vi "Parametric or Manual Arm Movement.vi"(0 "Desired Parametric\nValue":dbl, 1 "Forearm Manual\nControl":bool=TRUE, 2 "Change in\nForearm Angle":dbl, 5 "Current Parametric\nValue":dbl, 9 "Current Backarm\nAngle":dbl, 11 "Current Forearm\nAngle":dbl, 12 "Points":dbl[][](array[numeric]), 13 "Robot\nDimensions":cluster{}) -> (4 "New Backarm\nAngle":dbl, 6 "New Forearm\nAngle":dbl, 8 "Next Parametric\nValue":dbl, 10 "Apply Backarm\nBreak":bool=TRUE, 15 "Apply Forearm\nBreak":bool=TRUE)   [LabVIEW 2017]
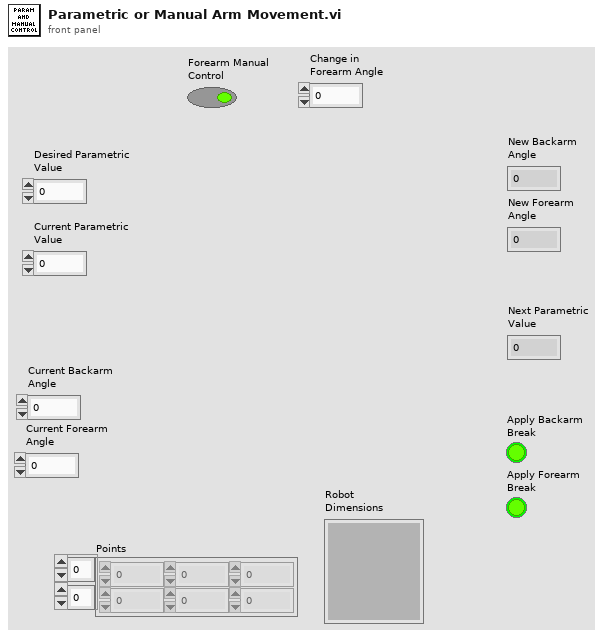
[diagram p1: front panel]
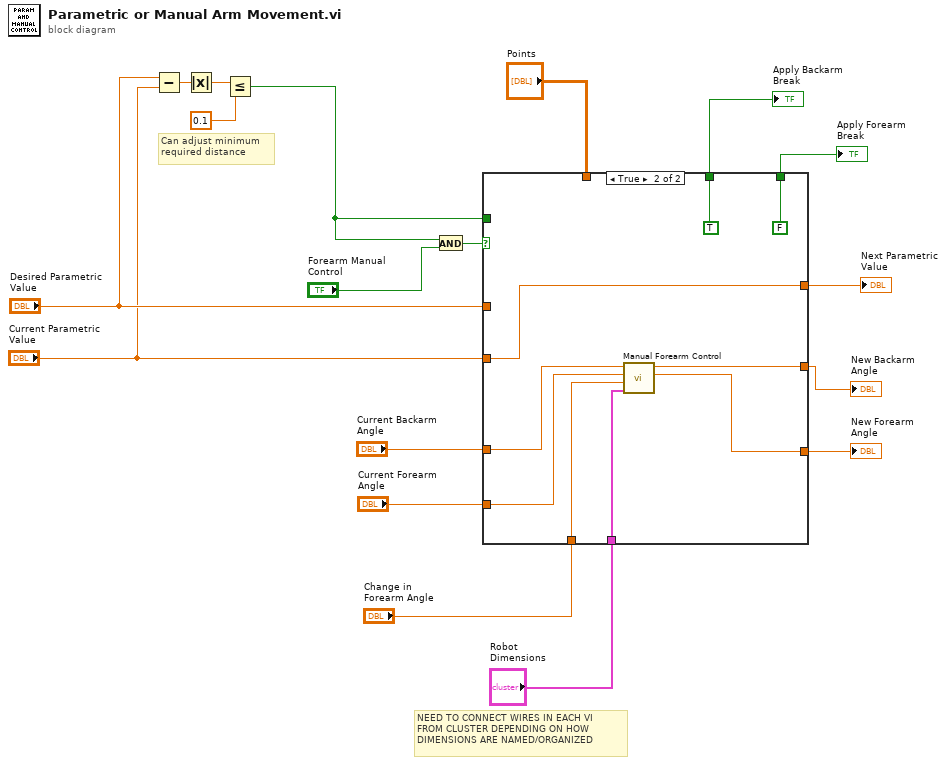
[diagram p0: block diagram]
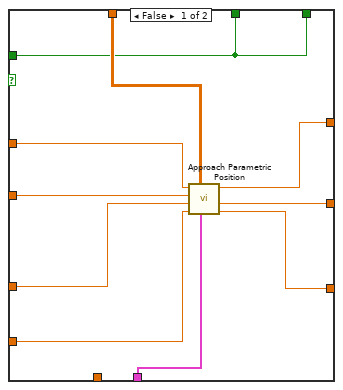
[diagram p2: hidden frame]
diagram:
  # "NEED TO CONNECT WIRES IN EACH VI\nFROM CLUSTER DEPENDING ON HOW \nDIMENSIONS ARE NAMED/ORGANIZED"
  # "Can adjust minimum\nrequired distance"
  n1 = Subtract(x="Desired Parametric\nValue", y="Current Parametric\nValue") -> (x-y=w9:dbl)
  n2 = Absolute Value(x=w9) -> (abs(x)=w8:dbl)
  n3 = Less Or Equal?(x=w8, y=0.1) -> (x <= y?=w3:bool)
  n4 = And(x=w3, y="Forearm Manual\nControl") -> (x .and. y?=w13:bool)
  n5 = case shown="True" w13 {
    tunnel: "Points" -> [w28 _]
    tunnel: "Current Parametric\nValue" -> [w27 w31]
    tunnel: "Desired Parametric\nValue" -> [w26 _]
    tunnel: "Current Backarm\nAngle" -> [w25 w36]
    tunnel: "Current Forearm\nAngle" -> [w24 w35]
    tunnel: [w23 w34] -> w15
    tunnel: [w22 w33] -> w14
    tunnel: "Robot\nDimensions" -> [w21 w37]
    tunnel: "Change in\nForearm Angle" -> [_ w32]
    tunnel: [w20 w31] -> w4
    tunnel: w3 -> [w19 _]
    tunnel: [w19 TRUE] -> w2
    tunnel: [w19 FALSE] -> w1
    frame False {
      n6 = call "Approach Parametric Position.vi"("Robot\nDimensions"=w21, "Points"=w28, "Initial Forearm\nAngle"=w24, "Initial Backarm\nAngle"=w25, "Initial Parametric\nValue"=w27, "New Parametric\nValue"=w26) -> ("Next Forearm\nAngle"=w22:dbl, "Next Backarm\nAngle"=w23:dbl, "Next Parametric\nValue"=w20:dbl)  [unwired: 3 in]
    }
    frame True {
      n7 = call "Manual Forearm Control.vi"("Robot Dimensions"=w37, "Forearm Angle\nChange"=w32, "Current Forearm\nAngle"=w35, "Current Backarm\nAngle"=w36) -> ("New Forearm\nAngle"=w33:dbl, "New Backarm\nAngle"=w34:dbl)  [unwired: 6 in]
    }
  }
  "New Backarm\nAngle" <- w15
  "New Forearm\nAngle" <- w14
  "Next Parametric\nValue" <- w4
  "Apply Backarm\nBreak" <- w2
  "Apply Forearm\nBreak" <- w1
